vi "19.5-iFIR Filter.vi"() -> ()   [LabVIEW 2020]
doc: "Uses the Median Filter VI to analyze pulses in the presence of noise. The example generates a pulse contaminated with Gaussian noise and applies a median filter. For comparison purposes, the VI computes the pulse parameters of the filtered pulse."
uses:
  <vilib>/Analysis/5stat.llb/RMS (DBL).vi
  <vilib>/Analysis/3filter.llb/FIR Narrowband Filter (DBL).vi
  <vilib>/Analysis/NI_AALBase.lvlib
  <vilib>/Analysis/NI_AALPro.lvlib
panel:
  out "Attenuation(dB)":dbl
  out "After Filter":dbl[](graph)
  in  "Filter Type":u32(ring) items=["Lowpass", "Highpass", "Bandpass", "Bandstop"]
  out "Before Filter":dbl[](graph)
  out "H[k]":dbl[](graph)
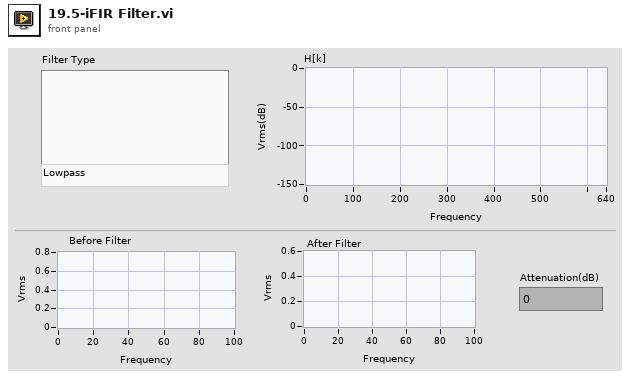
[diagram p1: front panel]
types:
  T1 = enum32{"Vrms", "Vpk", "Vrms^2", "Vpk^2", "Vrms/rtHz", "Vpk/rtHz", "Vrms^2/Hz", "Vpk^2/Hz"}
  T2 = enum16{"Power (Vrms^2)", "Amplitude (Vrms)", "Gain (amplitude ratio)"}
  T3 = cluster{"filter type":enum32{"Lowpass", "Highpass", "Bandpass", "Bandstop", "Wideband-Lowpass", "Wideband-Highpass"}, "interpolation":i32, "Model Filter":dbl[], "Image Suppressor":dbl[]}
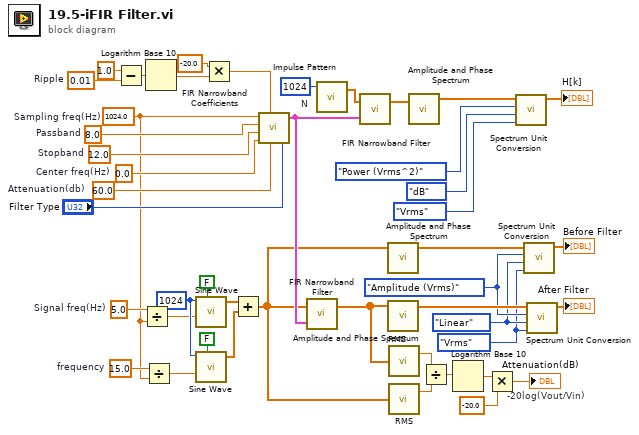
[diagram p0: block diagram]
diagram:
  w22 = 5.0  # Signal freq(Hz)
  w41 = 0.01  # Ripple
  w1 = 1024.0  # Sampling freq(Hz)
  w43 = 8.0  # Passband
  w44 = 12.0  # Stopband
  w45 = 0.0  # Center freq(Hz)
  w42 = 60.0  # Attenuation(db)
  w4 = T1."Vrms" ("display unit")
  w5 = enum16{"Linear", "dB", "dBm"}."Linear" ("log/linear")
  w6 = T2."Amplitude (Vrms)" ("spectrum type")
  w20 = 15.0  # frequency
  w23 = 1024 ("samples")
  w35 = 1024  # N
  # "-20log(Vout/Vin)"
  n1 = Subtract(x=1.0, y=w41) -> (x-y=w40:dbl)
  n2 = Divide(x=w22, y=w1) -> (x/y=w21:dbl)
  n3 = Divide(x=w20, y=w1) -> (x/y=w19:dbl)
  n4 = Logarithm Base 10(1:w40) -> (0:w38:dbl)
  n5 = call <vilib>:"Sine Wave.vi"("samples"=w23, "frequency"=w21, "reset phase"=FALSE) -> ("sine wave"=w18:dbl[])  [unwired: 2 in, 2 out]
  n6 = call <vilib>:"Sine Wave.vi"("samples"=w23, "frequency"=w19, "reset phase"=FALSE) -> ("sine wave"=w17:dbl[])  [unwired: 2 in, 2 out]
  n7 = Multiply(x=-20.0, y=w38) -> (x*y=w36:dbl)
  n8 = Add(x=w18, y=w17) -> (x+y=w3:dbl[])
  n9 = call <vilib>:"FIR Narrowband Coefficients.vi"("sampling freq: fs"=w1, "ripple: rp"=w36, "passband: fpass"=w43, "stopband: fstop"=w44, "attenuation (db): Ar"=w42, "center freq: fc"=w45, "filter type"="Filter Type") -> ("IFIR Coefficients"=w25:T3)  [unwired: 1 out]
  n10 = call-poly <vilib>:"FIR Narrowband Filter.vi"("IFIR Coefficients"=w25, "X"=w3) -> ("Filtered X"=w7:dbl[])  [unwired: 1 out]
  n11 = call <vilib>:"Impulse Pattern.vi"("samples"=w35) -> ("Impulse Pattern"=w34:dbl[])  [unwired: 2 in, 1 out]
  n12 = call-poly <vilib>:"FIR Narrowband Filter.vi"("IFIR Coefficients"=w25, "X"=w34) -> ("Filtered X"=w28:dbl[])  [unwired: 1 out]
  n13 = call <vilib>:"Amplitude and Phase Spectrum.vi"("Signal (V)"=w3) -> ("Amp Spectrum Mag (Vrms)"=w2:dbl[])  [unwired: 2 in, 2 out]
  n14 = call <vilib>:"Amplitude and Phase Spectrum.vi"("Signal (V)"=w7) -> ("Amp Spectrum Mag (Vrms)"=w16:dbl[])  [unwired: 2 in, 2 out]
  n15 = call-poly <vilib>:"RMS.vi"("X"=w7) -> ("rms value"=w11:dbl)  [unwired: 1 out]
  n16 = call-poly <vilib>:"RMS.vi"("X"=w3) -> ("rms value"=w15:dbl)  [unwired: 1 out]
  n17 = call <vilib>:"Amplitude and Phase Spectrum.vi"("Signal (V)"=w28) -> ("Amp Spectrum Mag (Vrms)"=w27:dbl[])  [unwired: 2 in, 2 out]
  n18 = Divide(x=w11, y=w15) -> (x/y=w14:dbl)
  n19 = Logarithm Base 10(1:w14) -> (0:w13:dbl)
  n20 = Multiply(x=w13, y=-20.0) -> (x*y=→"Attenuation(dB)":dbl)
  n21 = call <vilib>:"Spectrum Unit Conversion.vi"("display unit"=T1."Vrms", "log/linear"=enum16{"Linear", "dB", "dBm"}."dB", "spectrum type"=T2."Power (Vrms^2)", "Spectrum in"=w27) -> ("Spectrum out"=→"H[k]":dbl[])  [unwired: 6 in, 1 out]
  n22 = call <vilib>:"Spectrum Unit Conversion.vi"("display unit"=w4, "log/linear"=w5, "spectrum type"=w6, "Spectrum in"=w2) -> ("Spectrum out"=→"Before Filter":dbl[])  [unwired: 6 in, 1 out]
  n23 = call <vilib>:"Spectrum Unit Conversion.vi"("display unit"=w4, "log/linear"=w5, "spectrum type"=w6, "Spectrum in"=w16) -> ("Spectrum out"=→"After Filter":dbl[])  [unwired: 6 in, 1 out]
